vi "rdb_net_write.vi"(6 "timeout ms (10000)":i32=10000, 8 "error in (no error)":errorcluster, 10 "data in":string, 11 "conn in":refnum<k5>) -> (0 "error out":errorcluster, 2 "bytes written":i32, 3 "conn out":refnum<k5>)   [LabVIEW 2017]
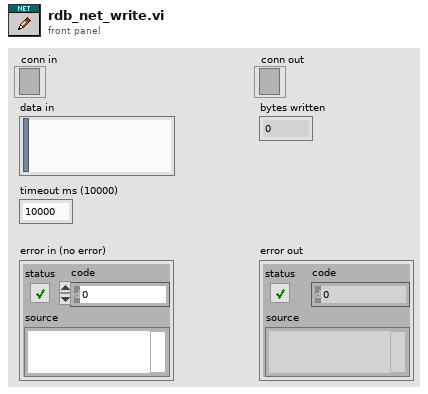
[diagram p1: front panel]
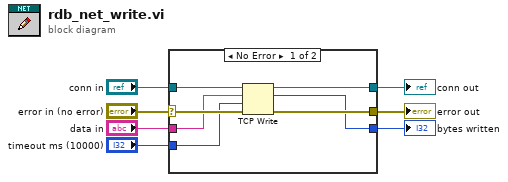
[diagram p0: block diagram]
diagram:
  n1 = case shown="No Error" "error in (no error)" {
    selector: "error in (no error)" -> [w14 w16]
    tunnel: [w13 w16] -> w6
    tunnel: "conn in" -> [w12 w15]
    tunnel: [w11 w15] -> w4
    tunnel: "timeout ms (10000)" -> [w10 _]
    tunnel: "data in" -> [w9 _]
    tunnel: [w8 _] -> w1
    frame No Error {
      n2 = TCP Write(connection ID=w12, data in=w9, error in (no error)=w14, 9:w10) -> (connection ID out=w11:refnum<k5>, bytes written=w8:i32, error out=w13:errorcluster)
    }
    frame Error {
    }
  }
  "error out" <- w6
  "conn out" <- w4
  "bytes written" <- w1
